vi "Close Module.vi"(8 "Error In":errorcluster) -> (0 "Error Out":errorcluster)   [LabVIEW 2023, in "Error Manager.lvlib" / "New Error Window.lvlib"]
uses:
  New Error Window.lvlib
  MHL Queue/Command (enum).ctl
  MHL Queue/MHL Queue.lvlib
panel:
  # "Development\ncontrols/indicators useful for development and testing, but which are not outputs of the VI"
  # "Input\nInputs to the VI"
  # "Output\nOutputs of the VI"
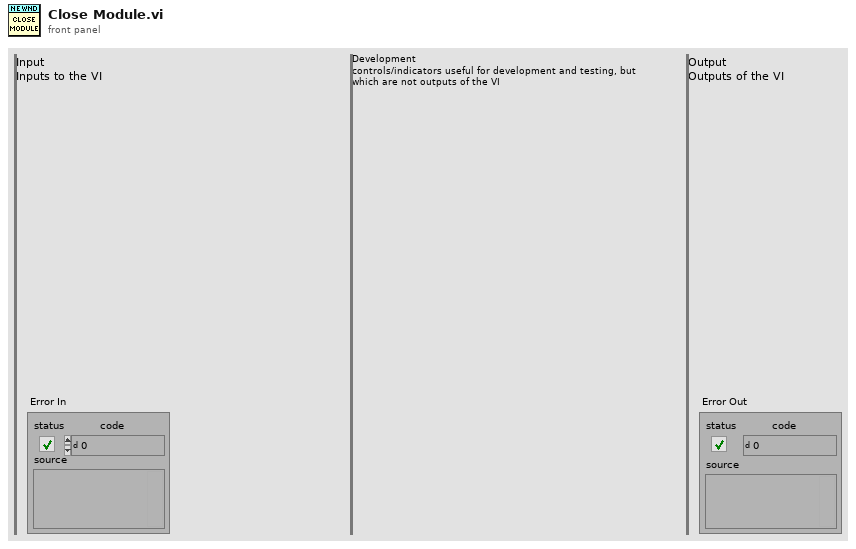
[diagram p1: front panel]
types:
  T1 = typedef "Error Manager.lvlib/New Error Window.lvlib/MHL Queue.lvlib/Command (enum).ctl" = enum16{"Init Module", "Close Module", "Handle Local Error", "OK Button Pressed"}
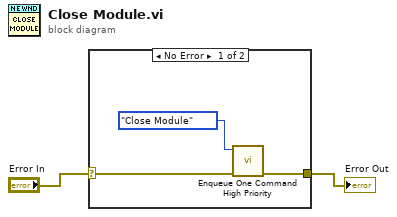
[diagram p0: block diagram]
diagram:
  n1 = case shown="No Error" "Error In" {
    selector: "Error In" -> [w4 w6]
    tunnel: [w3 w6] -> w1
    frame No Error {
      n2 = call "Enqueue One Command High Priority.vi"("error in (no error)"=w4, "Command"=Command_(enum)."Close Module") -> ("error out"=w3:errorcluster)  [unwired: 9 in]
    }
    frame Error {
    }
  }
  "Error Out" <- w1
